vi "DraadtoevoerMachine.vi"() -> ()   [LabVIEW 2013]
panel:
  in  "Tab Control":enum32{"Runtime operation", "Settings"}(tab)
  out "Wire Length [mm]":dbl(knob) scale=0.0..3150.0
  out "Spindle Speed [rad/s]":cluster{dbl, dbl}(knob)={0.0, 5.506200368166507} scale=0.01..5000.0
  out "Temperature log Next Spindle":dbl[](graph)
  out "Temperature log Current Spindle":dbl[](graph)
  in  "Emergency Button":bool
  out "SimulateWarning":string
  in  "Next spindle Type":string(combo)="Big 5[mm]"
  in  "Temperature set point [C]":dbl format="%#_3g"
  out "Next Spindel change [min]":cluster{dbl, dbl}(knob)={0.0, 7.436805212283668} scale=0.0..240.0
  in  "Current spindle Type":string(combo)="Big 5[mm]"
  in  "Temperature set point [C]":dbl format="%#_3g"
  out "Actual Temp next":dbl(slide) scale=0.0..100.0
  in  "Administrator password":string
  in  "stop":bool
  in  "Length set point [mm]":dbl=3000.0 format="%#_3g"
  out "Error Out":errorcluster
  in  "Min length alarm":dbl=30000.0
  in  "Temp low Deviation":dbl
  in  "Temp high Deviation":dbl
  in  "Run Simulation":bool=TRUE
  in  "DenProces 2":dbl[](array[numeric])
  in  "NumProcess 2":dbl[](array[numeric])
  in  "DenProces":dbl[](array[numeric])=[2.939e+25, 1.36e+27, 4.08e+27]
  in  "NumProcess":dbl[](array[numeric])=[0.0, 1.36e+27, 4.08e+27]
  # "Length Transfer Function"
  # "U"
  # "Omega"
  # "Heat Transfer Function"
  # "U"
  # "Temperature"
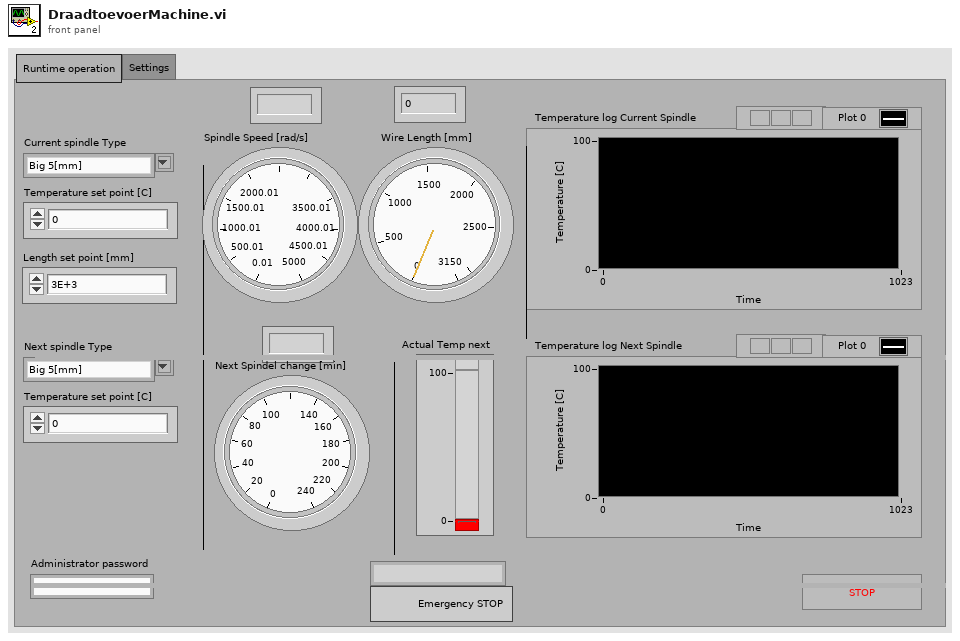
[diagram p1: front panel]
types:
  T1 = cluster{"Weight":dbl, "Radius":dbl, "Length":dbl}
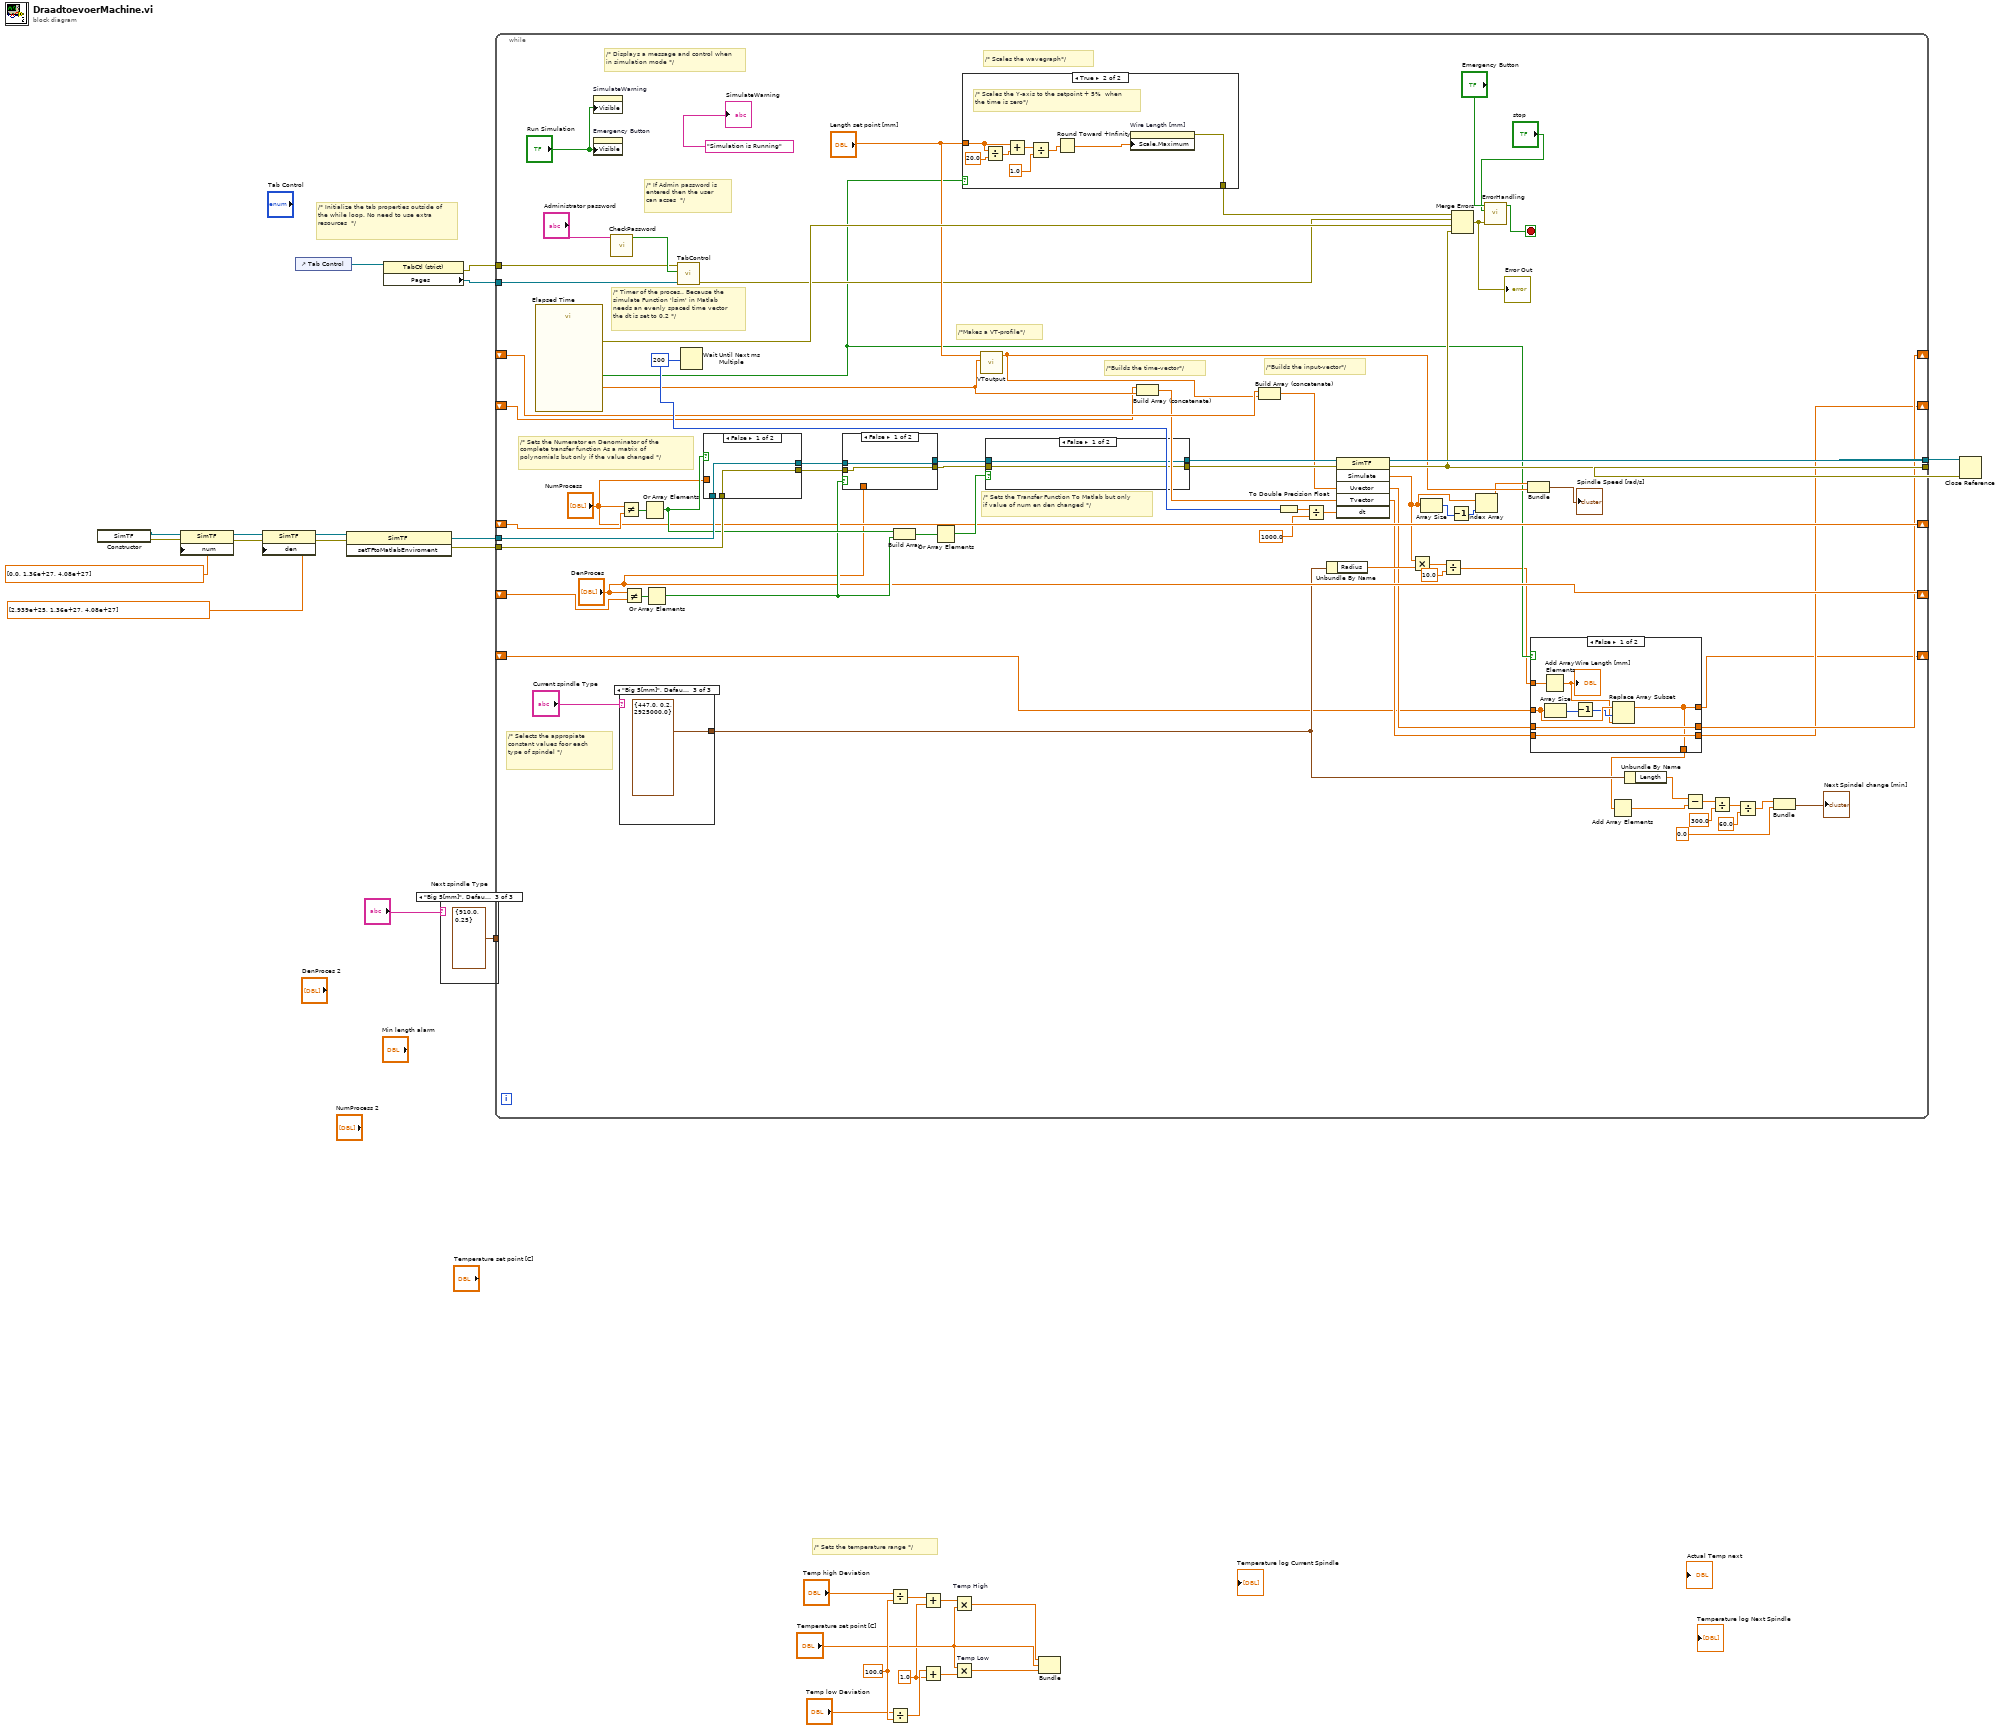
[diagram p0: block diagram]
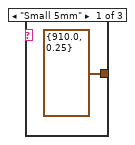
[diagram p2: hidden frame]
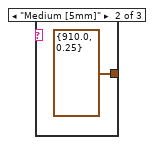
[diagram p3: hidden frame]
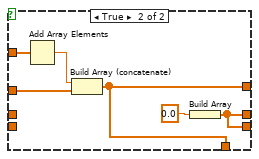
[diagram p4: hidden frame]
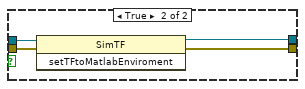
[diagram p6: hidden frame]
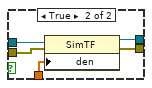
[diagram p7: hidden frame]
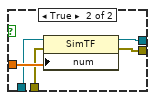
[diagram p8: hidden frame]
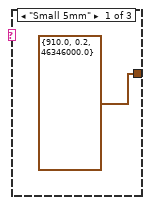
[diagram p9: hidden frame]
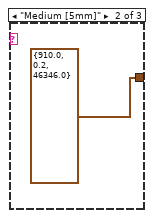
[diagram p10: hidden frame]
diagram:
  w23 = 100.0 ("y")
  w13 = 1.0 ("y")
  # "/* Sets the temperature range */"
  # "/* Initialize the tab properties outside of the while loop. No need to use extra resources  */"
  n1 = constructor class="SimTF"() -> (reference out=w8:refnum<k24>, error out=w7:errorcluster)  [unwired: 3 in, 1 out]
  n2 = property class="SimTF"(reference=w8, error in=w7, "num"=dbl[] [0.0, 1.36e+27, 4.08e+27]) -> (reference out=w10:refnum<k24>, error out=w9:errorcluster)
  n3 = property class="SimTF"(reference=w10, error in=w9, "den"=dbl[] [2.939e+25, 1.36e+27, 4.08e+27]) -> (reference out=w4:refnum<k24>, error out=w3:errorcluster)
  n4 = control-ref of="Tab Control"() -> (w27:refnum<vi>)
  n5 = invoke class="SimTF" method="setTFtoMatlabEnviroment"(reference=w4, error in=w3) -> (reference out=w2:refnum<k24>, error out=w1:errorcluster)  [unwired: 1 in, 1 out]
  n6 = property class="TabCtl (strict)"(reference=w27) -> (error out=w25:errorcluster, "Pages"=w26:refnum<vi>[])  [unwired: 1 in, 1 out]
  n7 = case shown="\"Big 5[mm]\", Default" "Next spindle Type" {
    tunnel: [cluster{"Weight":dbl, "Radius":dbl} {"Weight"=910.0, "Radius"=0.25} cluster{"Weight":dbl, "Radius":dbl} {"Weight"=910.0, "Radius"=0.25} cluster{"Weight":dbl, "Radius":dbl} {"Weight"=910.0, "Radius"=0.25}] -> _
    frame "Small 5mm" {
    }
    frame "Medium [5mm]" {
    }
    frame "Big 5[mm]", Default {
    }
  }
  n8 = while {
    tunnel: w26 -> [w93]
    tunnel: w1 -> [w88]
    tunnel: w2 -> [w87]
    tunnel: w25 -> [w92]
    tunnel: [w73] -> w24
    shift-right: ["NumProcess"] -> _
    shift-left: _ -> [w90]
    shift-right: ["DenProces"] -> _
    shift-left: _ -> [w86]
    tunnel: [w74] -> w11
    shift-right: [w48] -> _
    shift-left: _ -> [w63]
    shift-right: [w47] -> _
    shift-left: _ -> [w59]
    shift-right: [w38] -> _
    shift-left: _ -> [w37]
    stop <- w94 stop-if-true
    w65 = u32 200 ("millisecond multiple")
    # "/*Builds the input-vector*/"
    # "/*Builds the time-vector*/"
    # "/*Makes a VT-profile*/"
    # "/* Scales the wavegraph*/"
    # "/* Timer of the proces.. Because the simulate Function 'lsim' in Matlab needs an evenly spaced time vector the dt is set to 0.2 */"
    # "/* Sets the Transfer Function To Matlab but only if value of num en den changed */"
    # "/* If Admin password is entered then the user can acses  */"
    # "/* Sets the Numerator en Denominator of the complete transfer function As a matrix of polynomials but only if the value changed */"
    # "/* Displays a message and control when in simulation mode */"
    # "/* Selects the appropiate constant values foor each type of spindel */"
    n9 = call "Elapsed Time"() -> ("Elapsed Time (s)"=w62:dbl, "Time has Elapsed"=w53:bool, "error out"=w91:errorcluster)  [unwired: 12 in, 5 out]
    n10 = property on="SimulateWarning" class="Str"("Visible"="Run Simulation") -> ()  [unwired: 2 in, 2 out]
    n11 = property on="Emergency Button" class="Bool (strict)"("Visible"="Run Simulation") -> ()  [unwired: 2 in, 2 out]
    n12 = call "CheckPassword.vi"("Administrator password"="Administrator password") -> ("Boolean"=w99:bool)  [unwired: 10 in]
    n13 = Not Equal?(x="NumProcess", y=w90) -> (x != y?=w89:bool[])
    n14 = case shown="\"Big 5[mm]\", Default" "Current spindle Type" {
      tunnel: [T1 {"Weight"=910.0, "Radius"=0.2, "Length"=46346000.0} T1 {"Weight"=910.0, "Radius"=0.2, "Length"=46346.0} T1 {"Weight"=447.0, "Radius"=0.2, "Length"=2925000.0}] -> w43
      frame "Small 5mm" {
      }
      frame "Medium [5mm]" {
      }
      frame "Big 5[mm]", Default {
      }
    }
    n15 = Not Equal?(x="DenProces", y=w86) -> (x != y?=w85:bool[])
    n16 = Or Array Elements(Boolean array=w89) -> (logical OR=w79:bool)
    n17 = Or Array Elements(Boolean array=w85) -> (logical OR=w78:bool)
    n18 = call "TabControl.vi"("Pages"=w93, "Boolean"=w99, "error in (no error)"=w92) -> ("error out"=w71:errorcluster)  [unwired: 8 in]
    n19 = Wait Until Next ms Multiple(millisecond multiple=w65) -> ()  [unwired: 1 out]
    n20 = case shown="False" w79 {
      tunnel: w88 -> [w138 w140]
      tunnel: w87 -> [w139 w141]
      tunnel: [w139 w144] -> w84
      tunnel: [w138 w143] -> w83
      tunnel: "NumProcess" -> [_ w142]
      frame False {
      }
      frame True {
        n21 = property class="SimTF"(reference=w141, error in=w140, "num"=w142) -> (reference out=w144:refnum<k24>, error out=w143:errorcluster)
      }
    }
    n22 = case shown="False" w78 {
      tunnel: w84 -> [w132 w137]
      tunnel: w83 -> [w131 w136]
      tunnel: "DenProces" -> [_ w135]
      tunnel: [w132 w134] -> w82
      tunnel: [w131 w133] -> w81
      frame False {
      }
      frame True {
        n23 = property class="SimTF"(reference=w137, error in=w136, "den"=w135) -> (reference out=w134:refnum<k24>, error out=w133:errorcluster)
      }
    }
    n24 = Build Array(w79, w78) -> (w80:bool[])
    n25 = Or Array Elements(Boolean array=w80) -> (logical OR=w77:bool)
    n26 = case shown="True" w53 {
      tunnel: [_ w118] -> w70
      tunnel: "Length set point [mm]" -> [_ w124]
      frame False {
      }
      frame True {
        # "/* Scales the Y-axis to the setpoint + 5%  when the time is zero*/"
        n27 = Divide(x=w124, y=20.0) -> (x/y=w122:dbl)
        n28 = Add(x=w124, y=w122) -> (x+y=w121:dbl)
        n29 = Divide(x=w121, y=1.0) -> (x/y=w120:dbl)
        n30 = Round Toward +Infinity(x=w120) -> (ceil(x): smallest int >= x=w117:dbl)
        n31 = property on="Wire Length [mm]" class="Knob (strict)"("Scale.Maximum"=w117) -> (error out=w118:errorcluster)  [unwired: 2 in, 1 out]
      }
    }
    n32 = call "VToutput.vi"("Elapsed Time (s)"=w62, "Length set point [mm]"="Length set point [mm]") -> ("V"=w58:dbl)  [unwired: 9 in]
    n33 = case shown="False" w77 {
      tunnel: w82 -> [w126 w130]
      tunnel: w81 -> [w125 w129]
      tunnel: [w126 w128] -> w76
      tunnel: [w125 w127] -> w75
      frame False {
      }
      frame True {
        n34 = invoke class="SimTF" method="setTFtoMatlabEnviroment"(reference=w130, error in=w129) -> (reference out=w128:refnum<k24>, error out=w127:errorcluster)  [unwired: 1 in, 1 out]
      }
    }
    n35 = Build Array (concatenate)(w59, w62) -> (w60:dbl[])
    n36 = Build Array (concatenate)(w63, w58) -> (w61:dbl[])
    n37 = To Double Precision Float(number=w65) -> (double precision float=w66:dbl)
    n38 = Divide(x=w66, y=1000.0) -> (x/y=w67:dbl)
    n39 = Unbundle By Name(w43) -> ("Radius"=w52:dbl)
    n40 = invoke class="SimTF" method="Simulate"(reference=w76, error in=w75, "Uvector"=w61, "Tvector"=w60, "dt"=w67) -> (reference out=w74:refnum<k24>, error out=w73:errorcluster, "Simulate"=w51:dbl[], "Uvector"=w50:dbl[], "Tvector"=w49:dbl[])  [unwired: 1 in, 1 out]
    n41 = Multiply(x=w51, y=w52) -> (x*y=w46:dbl[])
    n42 = Array Size(array=w51) -> (size(s)=w55:i32)
    n43 = Divide(x=w46, y=10.0) -> (x/y=w45:dbl[])
    n44 = Decrement(x=w55) -> (x-1=w54:i32)
    n45 = Merge Errors(w70, w71, w91, w73) -> (w95:errorcluster)
    "Error Out" <- w95
    n46 = Index Array(array=w51, index=w54) -> (element=w57:dbl)
    n47 = call "ErrorHandling.vi"("error in (no error)"=w95, "stop"="stop", "Emergency Button"="Emergency Button") -> ("Boolean"=w94:bool)  [unwired: 8 in]
    n48 = Bundle(w57, "V"=w58) -> (→"Spindle Speed [rad/s]":cluster{dbl, "V":dbl})  [unwired: 1 in]
    n49 = case shown="False" w53 {
      tunnel: w45 -> [w108 w112]
      tunnel: w50 -> [w110 _]
      tunnel: w49 -> [w109 _]
      tunnel: [w110 w115] -> w48
      tunnel: [w109 w115] -> w47
      tunnel: [w103 w114] -> w39
      tunnel: [w103 w114] -> w38
      tunnel: w37 -> [w106 w113]
      frame False {
        n50 = Add Array Elements(numeric array=w108) -> (sum=w104:dbl)
        "Wire Length [mm]" <- w104
        n51 = Array Size(array=w106) -> (size(s)=w107:i32)
        n52 = Decrement(x=w107) -> (x-1=w105:i32)
        n53 = Replace Array Subset(array=w106, new element=w104, index=w105) -> (w103:dbl[])
      }
      frame True {
        n54 = Add Array Elements(numeric array=w112) -> (sum=w111:dbl)
        n55 = Build Array (concatenate)(w111, w113) -> (w114:dbl[])
        n56 = Build Array(0.0 ("element")) -> (w115:dbl[])
      }
    }
    n57 = Add Array Elements(numeric array=w39) -> (sum=w40:dbl)
    n58 = Unbundle By Name(w43) -> ("Length"=w42:dbl)
    n59 = Subtract(x=w42, y=w40) -> (x-y=w35:dbl)
    n60 = Divide(x=w35, y=300.0) -> (x/y=w33:dbl)
    n61 = Divide(x=w33, y=60.0) -> (x/y=w32:dbl)
    n62 = Bundle(w32, 0.0) -> (→"Next Spindel change [min]":cluster{dbl, dbl})  [unwired: 1 in]
    "SimulateWarning" <- "Simulation is Running" ("SimulateWarning")
  }
  n63 = Divide(x="Temp high Deviation", y=w23) -> (x/y=w19:dbl)
  n64 = Divide(x="Temp low Deviation", y=w23) -> (x/y=w21:dbl)
  n65 = Add(x=w19, y=w13) -> (x+y=w14:dbl)
  n66 = Add(x=w21, y=w13) -> (x+y=w15:dbl)
  n67 = Multiply "Temp High"(x=w14, y="Temperature set point [C]") -> (x*y=w16:dbl)
  n68 = Multiply "Temp Low"(x="Temperature set point [C]", y=w15) -> (x*y=w18:dbl)
  n69 = Bundle(w16, "Temperature set point [C]"="Temperature set point [C]", w18) -> ()  [unwired: 1 in, 1 out]
  n70 = Close Reference(reference=w11, error in (no error)=w24) -> ()  [unwired: 1 out]
